vi "BMU参数读取-Auto.vi"(7 "Socket":dbl, 8 "CAN端口":u16(ring), 9 "设备索引号":u16(ring), 10 "CAN卡类型":u32(ring)=21, 11 "从板号":u8=1) -> (3 "成功?":bool)   [LabVIEW 2013] (continued)
            }
          }
          event "DO1": Value Change {
            n4242 = event-data() -> ("NewVal"=w6074:bool)  [unwired: 6 out]
            n4243 = stacked-sequence {
              tunnel: w6074 -> [_ w6087 _]
              frame #0 {
                w6077 = FALSE ("清BUFF")
                n4244 = local write "继电器超时处理"(FALSE ("继电器超时处理")) -> ()
                n4245 = local write "清BUFF"(w6077) -> ()
                n4246 = local write "正级继电器 9"(w6077) -> ()
                n4247 = local write "主从选择"(enum32{"主板", "从板"}."主板" ("主从选择")) -> ()
              }
              frame #1 {
                n4248 = case shown="真" w6087 {
                  selector: w6087 -> [w6102 w6122]
                  tunnel: [w6101 w6121] -> w6086
                  tunnel: [w6089 w6109] -> w6081
                  frame False {
                    w6097 = 256.0 ("y")
                    w6089 = u32 2 ("命令序号")
                    w6101 = u8 192 ("命令")
                    n4249 = local read "动作保持时间"() -> (w6098:dbl)
                    n4250 = Quotient & Remainder(x=w6098, y=w6097) -> (x-y*floor(x/y)=w6090:dbl, floor(x/y)=w6094:dbl)
                    n4251 = Quotient & Remainder(x=w6094, y=w6097) -> (x-y*floor(x/y)=w6091:dbl, floor(x/y)=w6095:dbl)
                    n4252 = Quotient & Remainder(x=w6095, y=w6097) -> (x-y*floor(x/y)=w6092:dbl, floor(x/y)=w6096:dbl)
                    n4253 = local read "设备索引号"() -> (w6106:u16)
                    n4254 = local read "CAN卡类型"() -> (w6107:u32)
                    n4255 = local read "CAN端口"() -> (w6105:u16)
                    n4256 = Boolean To (0,1)(Boolean=w6102) -> (0, 1=w6099:i16)
                    n4257 = Quotient & Remainder(x=w6096, y=w6097) -> (x-y*floor(x/y)=w6093:dbl)  [unwired: 1 out]
                    n4258 = Build Array(i16 1 ("元素"), w6099, w6093, w6092, w6091, w6090, 0.0 ("元素")) -> (w6103:dbl[])
                    n4259 = call "多帧发送机制(EV05).vi"("can卡类型"=w6107, "设备索引号"=w6106, "CAN端口"=w6105, "命令"=w6101, "板号"=u8 0, "命令序号"=w6089, "输入数据"=w6103) -> ()  [unwired: 2 in, 11 out]
                  }
                  frame True {
                    w6117 = 256.0 ("y")
                    w6109 = u32 2 ("命令序号")
                    w6121 = u8 192 ("命令")
                    n4260 = local read "动作保持时间"() -> (w6118:dbl)
                    n4261 = Quotient & Remainder(x=w6118, y=w6117) -> (x-y*floor(x/y)=w6110:dbl, floor(x/y)=w6114:dbl)
                    n4262 = Quotient & Remainder(x=w6114, y=w6117) -> (x-y*floor(x/y)=w6111:dbl, floor(x/y)=w6115:dbl)
                    n4263 = Quotient & Remainder(x=w6115, y=w6117) -> (x-y*floor(x/y)=w6112:dbl, floor(x/y)=w6116:dbl)
                    n4264 = local read "设备索引号"() -> (w6126:u16)
                    n4265 = local read "CAN卡类型"() -> (w6127:u32)
                    n4266 = local read "CAN端口"() -> (w6125:u16)
                    n4267 = Boolean To (0,1)(Boolean=w6122) -> (0, 1=w6119:i16)
                    n4268 = Quotient & Remainder(x=w6116, y=w6117) -> (x-y*floor(x/y)=w6113:dbl)  [unwired: 1 out]
                    n4269 = Build Array(i16 1 ("元素"), w6119, w6113, w6112, w6111, w6110, 0.0 ("元素")) -> (w6123:dbl[])
                    n4270 = call "多帧发送机制(EV05).vi"("can卡类型"=w6127, "设备索引号"=w6126, "CAN端口"=w6125, "命令"=w6121, "板号"=u8 0, "命令序号"=w6109, "输入数据"=w6123) -> ()  [unwired: 2 in, 11 out]
                  }
                }
                n4271 = local write "命令序号"(w6081) -> ()
                n4272 = local write "命令"(w6086) -> ()
                n4273 = local write "控制1"(TRUE ("控制1")) -> ()
                n4274 = local write "写?"(FALSE ("写?")) -> ()
                n4275 = local write "消除"(TRUE ("消除")) -> ()
                n4276 = global write "EV05全局变量1.vi" "流控帧 2"(TRUE ("流控帧 2")) -> ()
                n4277 = global write "EV05全局变量1.vi" "流控帧"(FALSE ("流控帧")) -> ()
              }
              frame #2 {
                n4278 = flat-sequence {
                  tunnel: [w6129] -> w6128
                  tunnel: w6128 -> [w6136]
                  frame #0 {
                    n4279 = while {
                      tunnel: [w6130] -> w6129
                      i -> [w6134]
                      stop <- w6131 stop-if-true
                      n4280 = local read "继电器超时处理"() -> (w6130:bool)
                      n4281 = Greater Or Equal?(x=w6134, y=20) -> (x >= y?=w6132:bool)
                      n4282 = Wait Until Next ms Multiple(millisecond multiple=u32 100 ("毫秒倍数")) -> ()  [unwired: 1 out]
                      n4283 = Or(x=w6130, y=w6132) -> (x .or. y?=w6131:bool)
                    }
                  }
                  frame #1 {
                    n4284 = case shown="假" w6136 {
                      frame False {
                        n4285 = local read "DO1"() -> (w6138:bool)
                        n4286 = Not(x=w6138) -> (.not. x?=w6137:bool)
                        n4287 = local write "DO1"(w6137) -> ()
                        n4288 = One Button Dialog(message="DO控制处理超时" ("消息"), button name ("OK")="是" ("按钮名称（“确定”）")) -> ()  [unwired: 1 out]
                      }
                      frame True {
                      }
                    }
                  }
                }
              }
            }
          }
          event "DO2": Value Change {
            n4289 = event-data() -> ("NewVal"=w6141:bool)  [unwired: 6 out]
            n4290 = stacked-sequence {
              tunnel: w6141 -> [_ w6154 _]
              frame #0 {
                w6144 = FALSE ("清BUFF")
                n4291 = local write "继电器超时处理"(FALSE ("继电器超时处理")) -> ()
                n4292 = local write "主从选择"(enum32{"主板", "从板"}."主板" ("主从选择")) -> ()
                n4293 = local write "清BUFF"(w6144) -> ()
                n4294 = local write "正级继电器 10"(w6144) -> ()
              }
              frame #1 {
                n4295 = case shown="真" w6154 {
                  selector: w6154 -> [w6169 w6189]
                  tunnel: [w6168 w6188] -> w6153
                  tunnel: [w6156 w6176] -> w6148
                  frame False {
                    w6164 = 256.0 ("y")
                    w6156 = u32 2 ("命令序号")
                    w6168 = u8 192 ("命令")
                    n4296 = local read "动作保持时间"() -> (w6165:dbl)
                    n4297 = Quotient & Remainder(x=w6165, y=w6164) -> (x-y*floor(x/y)=w6157:dbl, floor(x/y)=w6161:dbl)
                    n4298 = Quotient & Remainder(x=w6161, y=w6164) -> (x-y*floor(x/y)=w6158:dbl, floor(x/y)=w6162:dbl)
                    n4299 = Quotient & Remainder(x=w6162, y=w6164) -> (x-y*floor(x/y)=w6159:dbl, floor(x/y)=w6163:dbl)
                    n4300 = local read "设备索引号"() -> (w6173:u16)
                    n4301 = local read "CAN卡类型"() -> (w6174:u32)
                    n4302 = local read "CAN端口"() -> (w6172:u16)
                    n4303 = Boolean To (0,1)(Boolean=w6169) -> (0, 1=w6166:i16)
                    n4304 = Quotient & Remainder(x=w6163, y=w6164) -> (x-y*floor(x/y)=w6160:dbl)  [unwired: 1 out]
                    n4305 = Build Array(i16 2 ("元素"), w6166, w6160, w6159, w6158, w6157, 0.0 ("元素")) -> (w6170:dbl[])
                    n4306 = call "多帧发送机制(EV05).vi"("can卡类型"=w6174, "设备索引号"=w6173, "CAN端口"=w6172, "命令"=w6168, "板号"=u8 0, "命令序号"=w6156, "输入数据"=w6170) -> ()  [unwired: 2 in, 11 out]
                  }
                  frame True {
                    w6184 = 256.0 ("y")
                    w6176 = u32 2 ("命令序号")
                    w6188 = u8 192 ("命令")
                    n4307 = local read "动作保持时间"() -> (w6185:dbl)
                    n4308 = Quotient & Remainder(x=w6185, y=w6184) -> (x-y*floor(x/y)=w6177:dbl, floor(x/y)=w6181:dbl)
                    n4309 = Quotient & Remainder(x=w6181, y=w6184) -> (x-y*floor(x/y)=w6178:dbl, floor(x/y)=w6182:dbl)
                    n4310 = Quotient & Remainder(x=w6182, y=w6184) -> (x-y*floor(x/y)=w6179:dbl, floor(x/y)=w6183:dbl)
                    n4311 = local read "设备索引号"() -> (w6193:u16)
                    n4312 = local read "CAN卡类型"() -> (w6194:u32)
                    n4313 = local read "CAN端口"() -> (w6192:u16)
                    n4314 = Boolean To (0,1)(Boolean=w6189) -> (0, 1=w6186:i16)
                    n4315 = Quotient & Remainder(x=w6183, y=w6184) -> (x-y*floor(x/y)=w6180:dbl)  [unwired: 1 out]
                    n4316 = Build Array(i16 2 ("元素"), w6186, w6180, w6179, w6178, w6177, 0.0 ("元素")) -> (w6190:dbl[])
                    n4317 = call "多帧发送机制(EV05).vi"("can卡类型"=w6194, "设备索引号"=w6193, "CAN端口"=w6192, "命令"=w6188, "板号"=u8 0, "命令序号"=w6176, "输入数据"=w6190) -> ()  [unwired: 2 in, 11 out]
                  }
                }
                n4318 = local write "命令序号"(w6148) -> ()
                n4319 = local write "命令"(w6153) -> ()
                n4320 = local write "控制1"(TRUE ("控制1")) -> ()
                n4321 = local write "写?"(FALSE ("写?")) -> ()
                n4322 = local write "消除"(TRUE ("消除")) -> ()
                n4323 = global write "EV05全局变量1.vi" "流控帧 2"(TRUE ("流控帧 2")) -> ()
                n4324 = global write "EV05全局变量1.vi" "流控帧"(FALSE ("流控帧")) -> ()
              }
              frame #2 {
                n4325 = flat-sequence {
                  tunnel: [w6196] -> w6195
                  tunnel: w6195 -> [w6203]
                  frame #0 {
                    n4326 = while {
                      tunnel: [w6197] -> w6196
                      i -> [w6201]
                      stop <- w6198 stop-if-true
                      n4327 = local read "继电器超时处理"() -> (w6197:bool)
                      n4328 = Greater Or Equal?(x=w6201, y=20) -> (x >= y?=w6199:bool)
                      n4329 = Wait Until Next ms Multiple(millisecond multiple=u32 100 ("毫秒倍数")) -> ()  [unwired: 1 out]
                      n4330 = Or(x=w6197, y=w6199) -> (x .or. y?=w6198:bool)
                    }
                  }
                  frame #1 {
                    n4331 = case shown="假" w6203 {
                      frame False {
                        n4332 = local read "DO2"() -> (w6205:bool)
                        n4333 = Not(x=w6205) -> (.not. x?=w6204:bool)
                        n4334 = local write "DO2"(w6204) -> ()
                        n4335 = One Button Dialog(message="DO控制处理超时" ("消息"), button name ("OK")="是" ("按钮名称（“确定”）")) -> ()  [unwired: 1 out]
                      }
                      frame True {
                      }
                    }
                  }
                }
              }
            }
          }
          event "DO1 2": Value Change {
            n4336 = event-data() -> ("NewVal"=w6208:bool)  [unwired: 6 out]
            n4337 = stacked-sequence {
              tunnel: w6208 -> [_ w6222 _]
              frame #0 {
                w6211 = FALSE ("继电器超时处理")
                n4338 = local write "继电器超时处理"(w6211) -> ()
                n4339 = local write "正级继电器 11"(w6211) -> ()
                n4340 = local write "主从选择"(enum32{"主板", "从板"}."从板" ("主从选择")) -> ()
              }
              frame #1 {
                n4341 = case shown="假" w6222 {
                  selector: w6222 -> [w6237 w6257]
                  tunnel: [w6236 w6256] -> w6221
                  tunnel: [w6235 w6255] -> w6215
                  tunnel: [w6224 w6244] -> w6216
                  frame True {
                    w6232 = 256.0 ("y")
                    w6224 = u32 2 ("命令序号")
                    w6236 = u8 192 ("命令")
                    n4342 = local read "动作保持时间"() -> (w6233:dbl)
                    n4343 = Quotient & Remainder(x=w6233, y=w6232) -> (x-y*floor(x/y)=w6225:dbl, floor(x/y)=w6229:dbl)
                    n4344 = Quotient & Remainder(x=w6229, y=w6232) -> (x-y*floor(x/y)=w6226:dbl, floor(x/y)=w6230:dbl)
                    n4345 = Quotient & Remainder(x=w6230, y=w6232) -> (x-y*floor(x/y)=w6227:dbl, floor(x/y)=w6231:dbl)
                    n4346 = Quotient & Remainder(x=w6231, y=w6232) -> (x-y*floor(x/y)=w6228:dbl)  [unwired: 1 out]
                    n4347 = Boolean To (0,1)(Boolean=w6237) -> (0, 1=w6234:i16)
                    n4348 = local read "设备索引号"() -> (w6241:u16)
                    n4349 = local read "CAN卡类型"() -> (w6242:u32)
                    n4350 = local read "从板板号"() -> (w6235:u8)
                    n4351 = local read "CAN端口"() -> (w6240:u16)
                    n4352 = Build Array(i16 3 ("元素"), w6234, w6228, w6227, w6226, w6225, 0.0 ("元素")) -> (w6239:dbl[])
                    n4353 = call "多帧发送机制(EV05).vi"("can卡类型"=w6242, "设备索引号"=w6241, "CAN端口"=w6240, "命令"=w6236, "板号"=w6235, "命令序号"=w6224, "输入数据"=w6239) -> ()  [unwired: 2 in, 11 out]
                  }
                  frame False {
                    w6252 = 256.0 ("y")
                    w6244 = u32 2 ("命令序号")
                    w6256 = u8 192 ("命令")
                    n4354 = local read "动作保持时间"() -> (w6253:dbl)
                    n4355 = Quotient & Remainder(x=w6253, y=w6252) -> (x-y*floor(x/y)=w6245:dbl, floor(x/y)=w6249:dbl)
                    n4356 = Quotient & Remainder(x=w6249, y=w6252) -> (x-y*floor(x/y)=w6246:dbl, floor(x/y)=w6250:dbl)
                    n4357 = Quotient & Remainder(x=w6250, y=w6252) -> (x-y*floor(x/y)=w6247:dbl, floor(x/y)=w6251:dbl)
                    n4358 = Quotient & Remainder(x=w6251, y=w6252) -> (x-y*floor(x/y)=w6248:dbl)  [unwired: 1 out]
                    n4359 = Boolean To (0,1)(Boolean=w6257) -> (0, 1=w6254:i16)
                    n4360 = local read "设备索引号"() -> (w6261:u16)
                    n4361 = local read "CAN卡类型"() -> (w6262:u32)
                    n4362 = local read "从板板号"() -> (w6255:u8)
                    n4363 = local read "CAN端口"() -> (w6260:u16)
                    n4364 = Build Array(i16 1 ("元素"), w6254, w6248, w6247, w6246, w6245, 0.0 ("元素")) -> (w6259:dbl[])
                    n4365 = call "多帧发送机制(EV05).vi"("can卡类型"=w6262, "设备索引号"=w6261, "CAN端口"=w6260, "命令"=w6256, "板号"=w6255, "命令序号"=w6244, "输入数据"=w6259) -> ()  [unwired: 2 in, 11 out]
                  }
                }
                n4366 = local write "从板板号"(w6215) -> ()
                n4367 = local write "命令序号"(w6216) -> ()
                n4368 = local write "命令"(w6221) -> ()
                n4369 = local write "清BUFF"(FALSE ("清BUFF")) -> ()
                n4370 = local write "写?"(FALSE ("写?")) -> ()
                n4371 = local write "控制1"(TRUE ("控制1")) -> ()
                n4372 = global write "EV05全局变量1.vi" "流控帧"(FALSE ("流控帧")) -> ()
                n4373 = global write "EV05全局变量1.vi" "流控帧 2"(TRUE ("流控帧 2")) -> ()
                n4374 = local write "消除"(TRUE ("消除")) -> ()
              }
              frame #2 {
                n4375 = flat-sequence {
                  tunnel: [w6264] -> w6263
                  tunnel: w6263 -> [w6271]
                  frame #0 {
                    n4376 = while {
                      tunnel: [w6265] -> w6264
                      i -> [w6269]
                      stop <- w6266 stop-if-true
                      n4377 = local read "继电器超时处理"() -> (w6265:bool)
                      n4378 = Greater Or Equal?(x=w6269, y=20) -> (x >= y?=w6267:bool)
                      n4379 = Wait Until Next ms Multiple(millisecond multiple=u32 100 ("毫秒倍数")) -> ()  [unwired: 1 out]
                      n4380 = Or(x=w6265, y=w6267) -> (x .or. y?=w6266:bool)
                    }
                  }
                  frame #1 {
                    n4381 = case shown="假" w6271 {
                      frame False {
                        n4382 = local read "DO1 2"() -> (w6273:bool)
                        n4383 = Not(x=w6273) -> (.not. x?=w6272:bool)
                        n4384 = local write "DO1 2"(w6272) -> ()
                        n4385 = One Button Dialog(message="DO控制处理超时" ("消息"), button name ("OK")="是" ("按钮名称（“确定”）")) -> ()  [unwired: 1 out]
                      }
                      frame True {
                      }
                    }
                  }
                }
              }
            }
          }
          event "读取转换为写入": Value Change {
            n4386 = event-data() -> ("NewVal"=w6276:bool)  [unwired: 6 out]
            n4387 = case shown="真" w6276 {
              tunnel: w6280 -> [w6282 w6287]
              tunnel: [w6282 w6286] -> w6279
              tunnel: w6278 -> [w6281 w6285]
              tunnel: [w6281 w6284] -> w6277
              frame False {
              }
              frame True {
                n4388 = Enqueue Element(queue=w6287, element="读取转换为写入", error in (no error)=w6285) -> (queue out=w6286:refnum<queue>, error out=w6284:errorcluster)  [unwired: 2 out]
              }
            }
          }
          event "读取故障详细状态": Value Change {
            n4389 = event-data() -> ("NewVal"=w6292:bool)  [unwired: 5 out]
            n4390 = case shown="真" w6292 {
              tunnel: w6291 -> [w6294 w6307]
              tunnel: w6290 -> [w6293 w6306]
              tunnel: [w6294 w6305] -> w6289
              tunnel: [w6293 w6304] -> w6288
              frame False {
              }
              frame True {
                n4391 = disable-structure shown="启用" {
                  disable-tunnel: [w6316 TRUE ("发送成功")] -> w6303
                  frame Disabled {
                    n4392 = local read "主从选择"() -> (w6308:enum32{"主板", "从板"})
                    n4393 = case shown="\"主板\", 默认" w6308 {
                      tunnel: [0.0 ("FUNC") w6318] -> w6313
                      frame "主板", Default {
                      }
                      frame "从板" {
                        n4394 = local read "从板号"() -> (w6318:u8)
                      }
                    }
                    n4395 = local read "设备索引号"() -> (w6310:u16)
                    n4396 = local read "CAN卡类型"() -> (w6311:u32)
                    n4397 = local read "CAN端口"() -> (w6309:u16)
                    n4398 = call "标定授权发送.vi"("CAN卡类型"=w6311, "解锁类型"=enum16{"读取", "写", "下载"}."写", "设备索引号"=w6310, "CAN端口"=w6309, "是否连接"=TRUE, "板选择"=0, "FUNC"=w6313) -> ("发送成功"=w6316:bool)  [unwired: 8 out]
                  }
                  frame Enabled {
                  }
                }
                n4399 = case shown="真" w6303 {
                  tunnel: w6307 -> [w6321 w6326]
                  tunnel: w6306 -> [w6320 w6325]
                  tunnel: [w6321 w6323] -> w6305
                  tunnel: [w6320 w6322] -> w6304
                  frame False {
                  }
                  frame True {
                    n4400 = Enqueue Element(queue=w6326, element="读取故障状态" ("元素"), error in (no error)=w6325) -> (queue out=w6323:refnum<queue>, error out=w6322:errorcluster)  [unwired: 2 out]
                  }
                }
                n4401 = local write "电池故障"(string[][] []) -> ()
                n4402 = global write "EV05全局变量1.vi" "流控帧 2"(TRUE ("流控帧")) -> ()
                n4403 = local write "写?"(FALSE ("写?")) -> ()
                n4404 = local write "控制1"(TRUE ("控制1")) -> ()
                n4405 = local write "消除"(TRUE ("消除")) -> ()
                n4406 = local write "清BUFF"(FALSE ("清BUFF")) -> ()
                n4407 = global write "EV05全局变量1.vi" "流控帧"(FALSE ("流控帧")) -> ()
                n4408 = call <vilib>:"Set Busy.vi"("disable click? (T)"=FALSE) -> ()  [unwired: 3 in, 8 out]
              }
            }
          }
          event "项目软本读取": Value Change {
            n4409 = event-data() -> ("NewVal"=w6331:bool)  [unwired: 5 out]
            n4410 = case shown="真" w6331 {
              tunnel: w6330 -> [w6333 w6338]
              tunnel: w6329 -> [w6332 w6337]
              tunnel: [w6333 w6336] -> w6328
              tunnel: [w6332 w6335] -> w6327
              frame False {
              }
              frame True {
                n4411 = stacked-sequence {
                  tunnel: [w6341] -> _
                  frame #0 {
                    w6341 = FALSE ("disable click? (T)")
                    w6344 = FALSE ("写?")
                    n4412 = local write "写?"(w6344) -> ()
                    n4413 = global write "EV05全局变量1.vi" "写入超时"(w6344) -> ()
                    n4414 = local write "项目软件版本号"(" " ("项目软件版本号")) -> ()
                    n4415 = global write "EV05全局变量1.vi" "流控帧"(FALSE ("流控帧")) -> ()
                    n4416 = local write "主从选择"(enum32{"主板", "从板"}."主板" ("主从选择")) -> ()
                    n4417 = call <vilib>:"Set Busy.vi"("disable click? (T)"=w6341) -> ()  [unwired: 3 in, 8 out]
                    n4418 = local write "清BUFF"(FALSE ("清BUFF")) -> ()
                    n4419 = property on="保存版本信息" class="Bool (严格)"("Visible"=TRUE ("可见")) -> ()  [unwired: 2 in, 2 out]
                    n4420 = global write "EV05全局变量1.vi" "流控帧 2"(TRUE ("流控帧 2")) -> ()
                    n4421 = local write "控制1"(TRUE ("控制1")) -> ()
                    n4422 = local write "消除"(TRUE ("消除")) -> ()
                  }
                }
                n4423 = Enqueue Element(queue=w6338, element="项目软件版本读取" ("元素"), error in (no error)=w6337) -> (queue out=w6336:refnum<queue>, error out=w6335:errorcluster)  [unwired: 2 out]
              }
            }
          }
          event "读硬件版本号": Value Change {
            n4424 = event-data() -> ("NewVal"=w6353:bool)  [unwired: 5 out]
            n4425 = case shown="真" w6353 {
              tunnel: w6352 -> [w6355 w6362]
              tunnel: w6351 -> [w6354 w6361]
              tunnel: [w6355 w6360] -> w6350
              tunnel: [w6354 w6359] -> w6349
              frame False {
              }
              frame True {
                n4426 = global read "EV05全局变量1.vi" "授权功能"() -> (w6357:bool)
                n4427 = case shown="真" w6357 {
                  tunnel: [TRUE ("发送成功") w6381] -> w6358
                  frame False {
                  }
                  frame True {
                    n4428 = local read "设备索引号"() -> (w6376:u16)
                    n4429 = local read "CAN卡类型"() -> (w6377:u32)
                    n4430 = local read "CAN端口"() -> (w6375:u16)
                    n4431 = call "标定授权发送.vi"("CAN卡类型"=w6377, "解锁类型"=enum16{"读取", "写", "下载"}."读取", "设备索引号"=w6376, "CAN端口"=w6375, "是否连接"=TRUE, "板选择"=0, "FUNC"=u32 0) -> ("发送成功"=w6381:bool)  [unwired: 8 in]
                  }
                }
                n4432 = stacked-sequence {
                  tunnel: [w6365] -> w6356
                  frame #0 {
                    w6365 = TRUE ("控制1")
                    w6369 = FALSE ("写?")
                    n4433 = local write "写?"(w6369) -> ()
                    n4434 = global write "EV05全局变量1.vi" "写入超时"(w6369) -> ()
                    n4435 = call <vilib>:"Set Busy.vi"("disable click? (T)"=FALSE) -> ()  [unwired: 3 in, 8 out]
                    n4436 = local write "硬件版本号"("" ("硬件版本号")) -> ()
                    n4437 = property on="保存版本信息" class="Bool (严格)"("Visible"=TRUE ("可见")) -> ()  [unwired: 2 in, 2 out]
                    n4438 = local write "主从选择"(enum32{"主板", "从板"}."主板" ("主从选择")) -> ()
                    n4439 = local write "控制1"(w6365) -> ()
                    n4440 = local write "清BUFF"(FALSE ("清BUFF")) -> ()
                    n4441 = global write "EV05全局变量1.vi" "流控帧 2"(TRUE ("流控帧 2")) -> ()
                    n4442 = local write "消除"(TRUE ("消除")) -> ()
                    n4443 = global write "EV05全局变量1.vi" "流控帧"(FALSE ("流控帧")) -> ()
                  }
                }
                n4444 = case shown="真" w6358 {
                  tunnel: w6362 -> [w6383 w6388]
                  tunnel: w6361 -> [w6382 w6387]
                  tunnel: [w6383 w6385] -> w6360
                  tunnel: [w6382 w6384] -> w6359
                  tunnel: w6356 -> [_ _]
                  frame False {
                  }
                  frame True {
                    n4445 = Enqueue Element(queue=w6388, element="硬件版本读取" ("元素"), error in (no error)=w6387) -> (queue out=w6385:refnum<queue>, error out=w6384:errorcluster)  [unwired: 2 out]
                  }
                }
              }
            }
          }
          event "平台软件版本读取": Value Change {
            n4446 = event-data() -> ("NewVal"=w6393:bool)  [unwired: 5 out]
            n4447 = case shown="真" w6393 {
              tunnel: w6392 -> [w6395 w6400]
              tunnel: w6391 -> [w6394 w6399]
              tunnel: [w6395 w6398] -> w6390
              tunnel: [w6394 w6397] -> w6389
              frame False {
              }
              frame True {
                n4448 = stacked-sequence {
                  tunnel: [w6403] -> _
                  frame #0 {
                    w6403 = TRUE ("控制1")
                    w6407 = FALSE ("写?")
                    n4449 = call <vilib>:"Set Busy.vi"("disable click? (T)"=FALSE) -> ()  [unwired: 3 in, 8 out]
                    n4450 = local write "写?"(w6407) -> ()
                    n4451 = global write "EV05全局变量1.vi" "写入超时"(w6407) -> ()
                    n4452 = local write "平台软件版本号"(" " ("平台软件版本号")) -> ()
                    n4453 = local write "控制1"(w6403) -> ()
                    n4454 = local write "消除"(TRUE ("消除")) -> ()
                    n4455 = property on="保存版本信息" class="Bool (严格)"("Visible"=TRUE ("可见")) -> ()  [unwired: 2 in, 2 out]
                    n4456 = global write "EV05全局变量1.vi" "流控帧 2"(TRUE ("流控帧 2")) -> ()
                    n4457 = local write "主从选择"(enum32{"主板", "从板"}."主板" ("主从选择")) -> ()
                    n4458 = local write "清BUFF"(FALSE ("清BUFF")) -> ()
                    n4459 = global write "EV05全局变量1.vi" "流控帧"(FALSE ("流控帧")) -> ()
                  }
                }
                n4460 = Enqueue Element(queue=w6400, element="平台软件版本读取" ("元素"), error in (no error)=w6399) -> (queue out=w6398:refnum<queue>, error out=w6397:errorcluster)  [unwired: 2 out]
              }
            }
          }
          event "模块版本读取": Value Change {
            n4461 = event-data() -> ("NewVal"=w6415:bool)  [unwired: 5 out]
            n4462 = case shown="真" w6415 {
              tunnel: w6414 -> [w6417 w6424]
              tunnel: w6413 -> [w6416 w6423]
              tunnel: [w6417 w6422] -> w6412
              tunnel: [w6416 w6421] -> w6411
              frame False {
              }
              frame True {
                n4463 = global read "EV05全局变量1.vi" "授权功能"() -> (w6419:bool)
                n4464 = case shown="假" w6419 {
                  tunnel: [TRUE ("发送成功") w6442] -> w6420
                  frame False {
                  }
                  frame True {
                    n4465 = local read "设备索引号"() -> (w6437:u16)
                    n4466 = local read "CAN卡类型"() -> (w6438:u32)
                    n4467 = local read "CAN端口"() -> (w6436:u16)
                    n4468 = call "标定授权发送.vi"("CAN卡类型"=w6438, "解锁类型"=enum16{"读取", "写", "下载"}."读取", "设备索引号"=w6437, "CAN端口"=w6436, "是否连接"=TRUE, "板选择"=0, "FUNC"=u32 0) -> ("发送成功"=w6442:bool)  [unwired: 8 out]
                  }
                }
                n4469 = stacked-sequence {
                  tunnel: [w6427] -> w6418
                  frame #0 {
                    w6427 = TRUE ("控制1")
                    w6430 = FALSE ("写?")
                    n4470 = call <vilib>:"Set Busy.vi"("disable click? (T)"=FALSE) -> ()  [unwired: 3 in, 8 out]
                    n4471 = local write "写?"(w6430) -> ()
                    n4472 = global write "EV05全局变量1.vi" "写入超时"(w6430) -> ()
                    n4473 = local write "主从选择"(enum32{"主板", "从板"}."主板" ("主从选择")) -> ()
                    n4474 = local write "清BUFF"(FALSE ("清BUFF")) -> ()
                    n4475 = property on="保存版本信息" class="Bool (严格)"("Visible"=TRUE ("可见")) -> ()  [unwired: 2 in, 2 out]
                    n4476 = global write "EV05全局变量1.vi" "流控帧 2"(TRUE ("流控帧 2")) -> ()
                    n4477 = local write "控制1"(w6427) -> ()
                    n4478 = local write "消除"(TRUE ("消除")) -> ()
                    n4479 = global write "EV05全局变量1.vi" "流控帧"(FALSE ("流控帧")) -> ()
                  }
                }
                n4480 = case shown="真" w6420 {
                  tunnel: w6424 -> [w6444 w6449]
                  tunnel: w6423 -> [w6443 w6448]
                  tunnel: [w6444 w6446] -> w6422
                  tunnel: [w6443 w6445] -> w6421
                  tunnel: w6418 -> [_ _]
                  frame False {
                  }
                  frame True {
                    n4481 = Enqueue Element(queue=w6449, element="模块软件版本读取" ("元素"), error in (no error)=w6448) -> (queue out=w6446:refnum<queue>, error out=w6445:errorcluster)  [unwired: 2 out]
                  }
                }
              }
            }
          }
          event "保存版本信息": Value Change {
            n4482 = event-data() -> ("NewVal"=w6450:bool)  [unwired: 6 out]
            n4483 = case shown="真" w6450 {
              frame False {
              }
              frame True {
                n4484 = stacked-sequence {
                  seq-local: [w6454 _] -> [_ w6456]
                  seq-local: [w6453 _] -> [_ w6455]
                  frame #0 {
                    n4485 = call "请输入从板个数"() -> ("从板个数"=w6454:dbl, "确定"=w6453:bool)  [unwired: 17 in, 1 out]
                  }
                  frame #1 {
                    n4486 = case shown="真" w6455 {
                      tunnel: w6456 -> [_ w6459]
                      frame False {
                      }
                      frame True {
                        n4487 = call <vilib>:"Application Directory.vi"() -> ("Application Directory"=w6471:path)
                        n4488 = Build Path(base path=w6471, name or relative path="SaveData" ("名称或相对路径")) -> (appended path=w6469:path)
                        n4489 = local read "模块版本名称"() -> (w6464:string[][])
                        n4490 = local read "项目软件版本"() -> (w6461:string[])
                        n4491 = local read "模块版本值"() -> (w6463:string[][])
                        n4492 = local read "平台软件版本"() -> (w6460:string[])
                        n4493 = local read "模块个数"() -> (w6457:u8[])
                        n4494 = local read "硬件版本"() -> (w6462:string[])
                        n4495 = call "文件对话框3"("start path"=w6469, "prompt"="选择要保存数据的位置", "default name"="BMS版本信息.txt") -> ("selected path"=w6465:path, "cancelled"=w6466:bool)  [unwired: 9 in, 2 out]
                        n4496 = Increment(x=w6459) -> (x+1=w6458:dbl)
                        n4497 = for {
                          N: w6458 -> [_]
                          tunnel: w6466 -> [w6487]
                          tunnel: w6465 -> [w6486]
                          tunnel: w6464 -> [w6476] mode=indexing
                          tunnel: w6463 -> [w6474] mode=indexing
                          tunnel: w6462 -> [w6481] mode=indexing
                          tunnel: w6461 -> [w6480] mode=indexing
                          tunnel: w6460 -> [w6479] mode=indexing
                          tunnel: w6457 -> [w6472] mode=indexing
                          i -> [w6478]
                          w6484 = ""
                          w6491 = 0 ("索引")
                          n4498 = case shown="0, 默认" w6478 {
                            selector: w6478 -> [_ w6505]
                            tunnel: ["主板版本信息" w6506] -> w6496
                            tunnel: [FALSE TRUE] -> w6482
                            frame 0, Default {
                            }
                            frame 1.. {
                              n4499 = Number To Decimal String(number=w6505) -> (decimal integer string=w6504:string)  [unwired: 1 in]
                              n4500 = Concatenate Strings("从板", w6504, "版本信息") -> (w6506:string)
                            }
                          }
                          n4501 = Increment(x=w6472) -> (x+1=w6473:u8)
                          n4502 = Array Subset(array=w6476, length=w6473) -> (w6477:string[])  [unwired: 1 in]
                          n4503 = Array Subset(array=w6474, length=w6473) -> (w6475:string[])  [unwired: 1 in]
                          n4504 = Build Array(w6484, w6479, w6480, w6481, w6484) -> (w6490:string[])
                          n4505 = Build Array(w6496, "平台软件版本号", "项目软件版本号", "硬件版本号", "模块版本号") -> (w6492:string[])
                          n4506 = Insert Into Array(array=w6477, index=w6491, new element=w6492) -> (w6489:string[])
                          n4507 = Insert Into Array(array=w6475, index=w6491, new element=w6490) -> (w6488:string[])
                          n4508 = Build Array(w6489, w6488) -> (w6485:string[][])
                          n4509 = case shown="假" w6487 {
                            tunnel: w6486 -> [w6500 _]
                            tunnel: w6485 -> [w6499 _]
                            tunnel: w6482 -> [w6497 _]
                            frame False {
                              n4510 = call-poly <vilib>:"Write To Spreadsheet File.vi"("transpose? (no:F)"=TRUE, "append to file? (new file:F)"=w6497, "2D data"=w6499, "file path (dialog if empty)"=w6500) -> ()  [unwired: 4 in, 1 out]
                            }
                            frame True {
                            }
                          }
                        }
                      }
                    }
                  }
                }
              }
            }
          }
          event "单个写入": Value Change {
            n4511 = event-data() -> ("NewVal"=w6513:bool)  [unwired: 5 out]
            n4512 = case shown="真" w6513 {
              tunnel: w6512 -> [w6515 w6522]
              tunnel: w6511 -> [w6514 w6521]
              tunnel: [w6515 w6520] -> w6510
              tunnel: [w6514 w6519] -> w6509
              frame False {
              }
              frame True {
                w6517 = FALSE ("流控帧")
                w6516 = TRUE ("流控帧 2")
                n4513 = disable-structure shown="禁用" {
                  disable-tunnel: [w6531 TRUE ("发送成功")] -> w6518
                  frame Disabled {
                    n4514 = local read "主从选择"() -> (w6523:enum32{"主板", "从板"})
                    n4515 = case shown="\"主板\", 默认" w6523 {
                      tunnel: [0.0 ("FUNC") w6533] -> w6528
                      frame "主板", Default {
                      }
                      frame "从板" {
                        n4516 = local read "从板号"() -> (w6533:u8)
                      }
                    }
                    n4517 = local read "设备索引号"() -> (w6525:u16)
                    n4518 = local read "CAN卡类型"() -> (w6526:u32)
                    n4519 = local read "CAN端口"() -> (w6524:u16)
                    n4520 = call "标定授权发送.vi"("CAN卡类型"=w6526, "解锁类型"=enum16{"读取", "写", "下载"}."写", "设备索引号"=w6525, "CAN端口"=w6524, "是否连接"=TRUE, "板选择"=0, "FUNC"=w6528) -> ("发送成功"=w6531:bool)  [unwired: 8 out]
                  }
                  frame Enabled {
                  }
                }
                n4521 = case shown="真" w6518 {
                  tunnel: w6522 -> [w6536 w6540]
                  tunnel: w6521 -> [w6535 w6539]
                  tunnel: [w6536 w6542] -> w6520
                  tunnel: [w6535 w6541] -> w6519
                  frame False {
                  }
                  frame True {
                    n4522 = Flush Queue(queue=w6540, error in (no error)=w6539) -> (queue out=w6538:refnum<queue>, error out=w6537:errorcluster)  [unwired: 1 out]
                    n4523 = Enqueue Element(queue=w6538, element="单个写入" ("元素"), error in (no error)=w6537) -> (queue out=w6542:refnum<queue>, error out=w6541:errorcluster)  [unwired: 2 out]
                  }
                }
                n4524 = global write "EV05全局变量1.vi" "读取超时"(w6517) -> ()
                n4525 = global write "EV05全局变量1.vi" "流控帧"(w6517) -> ()
                n4526 = local write "消除"(w6516) -> ()
                n4527 = local write "控制1"(w6516) -> ()
                n4528 = global write "EV05全局变量1.vi" "流控帧 2"(w6516) -> ()
                n4529 = local write "写?"(w6516) -> ()
              }
            }
          }
          event "全部写入": Value Change {
            n4530 = event-data() -> ("NewVal"=w6548:bool)  [unwired: 5 out]
            n4531 = case shown="真" w6548 {
              tunnel: w6547 -> [w6550 w6558]
              tunnel: w6546 -> [w6549 w6557]
              tunnel: [w6550 w6556] -> w6545
              tunnel: [w6549 w6555] -> w6544
              frame False {
              }
              frame True {
                w6552 = FALSE ("流控帧")
                w6551 = TRUE ("流控帧 2")
                n4532 = global read "EV05全局变量1.vi" "授权功能"() -> (w6553:bool)
                n4533 = case shown="真" w6553 {
                  tunnel: [TRUE ("发送成功") w6568] -> w6554
                  frame False {
                  }
                  frame True {
                    n4534 = local read "主从选择"() -> (w6560:enum32{"主板", "从板"})
                    n4535 = case shown="\"从板\"" w6560 {
                      tunnel: [0.0 ("FUNC") w6570] -> w6561
                      frame "主板", Default {
                      }
                      frame "从板" {
                        n4536 = local read "从板号"() -> (w6570:u8)
                      }
                    }
                    n4537 = local read "设备索引号"() -> (w6563:u16)
                    n4538 = local read "CAN卡类型"() -> (w6564:u32)
                    n4539 = local read "CAN端口"() -> (w6562:u16)
                    n4540 = call "标定授权发送.vi"("CAN卡类型"=w6564, "解锁类型"=enum16{"读取", "写", "下载"}."写", "设备索引号"=w6563, "CAN端口"=w6562, "是否连接"=TRUE, "板选择"=0, "FUNC"=w6561) -> ("发送成功"=w6568:bool)  [unwired: 8 out]
                  }
                }
                n4541 = case shown="真" w6554 {
                  tunnel: w6558 -> [w6572 w6576]
                  tunnel: w6557 -> [w6571 w6575]
                  tunnel: [w6572 w6578] -> w6556
                  tunnel: [w6571 w6577] -> w6555
                  frame False {
                  }
                  frame True {
                    n4542 = Flush Queue(queue=w6576, error in (no error)=w6575) -> (queue out=w6574:refnum<queue>, error out=w6573:errorcluster)  [unwired: 1 out]
                    n4543 = Enqueue Element(queue=w6574, element="全部写入" ("元素"), error in (no error)=w6573) -> (queue out=w6578:refnum<queue>, error out=w6577:errorcluster)  [unwired: 1 in, 1 out]
                  }
                }
                n4544 = global write "EV05全局变量1.vi" "读取超时"(w6552) -> ()
                n4545 = global write "EV05全局变量1.vi" "流控帧"(w6552) -> ()
                n4546 = local write "消除"(w6551) -> ()
                n4547 = local write "控制1"(w6551) -> ()
                n4548 = global write "EV05全局变量1.vi" "流控帧 2"(w6551) -> ()
                n4549 = local write "写?"(w6551) -> ()
              }
            }
          }
          event "单个读取": Value Change {
            n4550 = event-data() -> ("NewVal"=w6584:bool)  [unwired: 5 out]
            n4551 = case shown="真" w6584 {
              tunnel: w6583 -> [w6586 w6594]
              tunnel: w6582 -> [w6585 w6593]
              tunnel: [w6586 w6592] -> w6581
              tunnel: [w6585 w6591] -> w6580
              frame False {
              }
              frame True {
                w6587 = FALSE ("流控帧")
                w6588 = TRUE ("流控帧 2")
                n4552 = global read "EV05全局变量1.vi" "授权功能"() -> (w6589:bool)
                n4553 = case shown="假" w6589 {
                  tunnel: [TRUE ("发送成功") w6603] -> w6590
                  frame False {
                  }
                  frame True {
                    n4554 = local read "设备索引号"() -> (w6597:u16)
                    n4555 = local read "CAN卡类型"() -> (w6598:u32)
                    n4556 = local read "CAN端口"() -> (w6596:u16)
                    n4557 = call "标定授权发送.vi"("CAN卡类型"=w6598, "解锁类型"=enum16{"读取", "写", "下载"}."读取", "设备索引号"=w6597, "CAN端口"=w6596, "是否连接"=TRUE, "板选择"=0, "FUNC"=u32 1) -> ("发送成功"=w6603:bool)  [unwired: 8 out]
                  }
                }
                n4558 = case shown="真" w6590 {
                  tunnel: w6594 -> [w6605 w6609]
                  tunnel: w6593 -> [w6604 w6607]
                  tunnel: [w6605 w6611] -> w6592
                  tunnel: [w6604 w6610] -> w6591
                  frame False {
                  }
                  frame True {
                    n4559 = Flush Queue(queue=w6609, error in (no error)=w6607) -> (queue out=w6608:refnum<queue>, error out=w6606:errorcluster)  [unwired: 1 out]
                    n4560 = Enqueue Element(queue=w6608, element="单个读取" ("元素"), error in (no error)=w6606) -> (queue out=w6611:refnum<queue>, error out=w6610:errorcluster)  [unwired: 2 out]
                  }
                }
                n4561 = global write "EV05全局变量1.vi" "写入超时"(w6587) -> ()
                n4562 = global write "EV05全局变量1.vi" "流控帧"(w6587) -> ()
                n4563 = local write "写?"(w6587) -> ()
                n4564 = local write "消除"(w6588) -> ()
                n4565 = local write "控制1"(w6588) -> ()
                n4566 = global write "EV05全局变量1.vi" "流控帧 2"(w6588) -> ()
              }
            }
          }
          event "全部读取": Value Change {
            n4567 = event-data() -> ("NewVal"=w6617:bool)  [unwired: 5 out]
            n4568 = case shown="真" w6617 {
              tunnel: w6616 -> [w6619 w6623]
              tunnel: w6615 -> [w6618 w6622]
              tunnel: [w6619 w6621] -> w6614
              tunnel: [w6618 w6620] -> w6613
              frame False {
              }
              frame True {
                n4569 = stacked-sequence {
                  seq-local: [w6628 _] -> [_ _]
                  seq-local: [w6627 _] -> [_ _]
                  tunnel: w6623 -> [w6630 w6659]
                  tunnel: w6622 -> [w6629 w6658]
                  tunnel: [_ w6663] -> w6621
                  tunnel: [_ w6662] -> w6620
                  frame #0 {
                    w6624 = FALSE ("布尔")
                    n4570 = local read "路径"() -> (w6626:path)
                    n4571 = Empty String/Path?(string/path=w6626) -> (empty?=w6625:bool)
                    n4572 = case shown="假" w6625 {
                      tunnel: w6630 -> [w6637 w6655]
                      tunnel: w6629 -> [w6636 w6654]
                      tunnel: [w6633 w6654] -> w6628
                      tunnel: [w6632 w6655] -> w6627
                      frame False {
                        n4573 = global read "EV05全局变量1.vi" "授权功能"() -> (w6634:bool)
                        n4574 = case shown="真" w6634 {
                          tunnel: [TRUE ("发送成功") w6646] -> w6635
                          frame False {
                          }
                          frame True {
                            n4575 = local read "设备索引号"() -> (w6640:u16)
                            n4576 = local read "CAN卡类型"() -> (w6641:u32)
                            n4577 = local read "CAN端口"() -> (w6639:u16)
                            n4578 = call "标定授权发送.vi"("CAN卡类型"=w6641, "解锁类型"=enum16{"读取", "写", "下载"}."读取", "设备索引号"=w6640, "CAN端口"=w6639, "是否连接"=TRUE, "板选择"=0, "FUNC"=u32 1) -> ("发送成功"=w6646:bool)  [unwired: 8 out]
                          }
                        }
                        n4579 = case shown="真" w6635 {
                          tunnel: w6637 -> [w6648 w6653]
                          tunnel: w6636 -> [w6647 w6652]
                          tunnel: [w6648 w6650] -> w6632
                          tunnel: [w6647 w6649] -> w6633
                          frame False {
                          }
                          frame True {
                            n4580 = Enqueue Element(queue=w6653, element="读配置文件" ("元素"), error in (no error)=w6652) -> (queue out=w6650:refnum<queue>, error out=w6649:errorcluster)  [unwired: 2 out]
                          }
                        }
                        n4581 = Wait Until Next ms Multiple(millisecond multiple=u32 200 ("毫秒倍数")) -> ()  [unwired: 1 out]
                      }
                      frame True {
                      }
                    }
                    n4582 = local write "1 6"(w6624) -> ()
                    n4583 = local write "1 7"(w6624) -> ()
                    n4584 = local write "1 8"(w6624) -> ()
                    n4585 = local write "1 9"(w6624) -> ()
                    n4586 = local write "1 10"(w6624) -> ()
                    n4587 = local write "1 12"(w6624) -> ()
                  }
                  frame #1 {
                    w6656 = FALSE ("流控帧")
                    w6657 = TRUE ("流控帧 2")
                    n4588 = global read "EV05全局变量1.vi" "授权功能"() -> (w6660:bool)
                    n4589 = case shown="假" w6660 {
                      tunnel: [TRUE ("发送成功") w6672] -> w6661
                      frame False {
                      }
                      frame True {
                        n4590 = local read "设备索引号"() -> (w6666:u16)
                        n4591 = local read "CAN卡类型"() -> (w6667:u32)
                        n4592 = local read "CAN端口"() -> (w6665:u16)
                        n4593 = call "标定授权发送.vi"("CAN卡类型"=w6667, "解锁类型"=enum16{"读取", "写", "下载"}."读取", "设备索引号"=w6666, "CAN端口"=w6665, "是否连接"=TRUE, "板选择"=0, "FUNC"=u32 1) -> ("发送成功"=w6672:bool)  [unwired: 8 out]
                      }
                    }
                    n4594 = case shown="真" w6661 {
                      tunnel: w6659 -> [w6674 w6675]
                      tunnel: w6658 -> [w6673 w6678]
                      tunnel: [w6674 w6680] -> w6663
                      tunnel: [w6673 w6679] -> w6662
                      frame False {
                      }
                      frame True {
                        n4595 = Flush Queue(queue=w6675, error in (no error)=w6678) -> (queue out=w6676:refnum<queue>, error out=w6677:errorcluster)  [unwired: 1 out]
                        n4596 = Enqueue Element(queue=w6676, element="全部读取" ("元素"), error in (no error)=w6677) -> (queue out=w6680:refnum<queue>, error out=w6679:errorcluster)  [unwired: 2 out]
                      }
                    }
                    n4597 = global write "EV05全局变量1.vi" "写入超时"(w6656) -> ()
                    n4598 = global write "EV05全局变量1.vi" "流控帧"(w6656) -> ()
                    n4599 = local write "写?"(w6656) -> ()
                    n4600 = local write "消除"(w6657) -> ()
                    n4601 = local write "控制1"(w6657) -> ()
                    n4602 = global write "EV05全局变量1.vi" "流控帧 2"(w6657) -> ()
                  }
                }
              }
            }
          }
          event "开启均衡": Value Change {
            n4603 = event-data() -> ("NewVal"=w6686:bool)  [unwired: 5 out]
            n4604 = case shown="真" w6686 {
              tunnel: w6685 -> [w6688 w6695]
              tunnel: w6684 -> [w6687 w6694]
              tunnel: [w6688 w6693] -> w6683
              tunnel: [w6687 w6692] -> w6682
              frame False {
              }
              frame True {
                n4605 = global read "EV05全局变量1.vi" "授权功能"() -> (w6690:bool)
                n4606 = case shown="假" w6690 {
                  tunnel: [TRUE ("发送成功") w6705] -> w6691
                  frame False {
                  }
                  frame True {
                    n4607 = local read "主从选择"() -> (w6697:enum32{"主板", "从板"})
                    n4608 = case shown="\"从板\"" w6697 {
                      tunnel: [0.0 ("FUNC") w6707] -> w6698
                      frame "主板", Default {
                      }
                      frame "从板" {
                        n4609 = local read "从板号"() -> (w6707:u8)
                      }
                    }
                    n4610 = local read "设备索引号"() -> (w6700:u16)
                    n4611 = local read "CAN卡类型"() -> (w6701:u32)
                    n4612 = local read "CAN端口"() -> (w6699:u16)
                    n4613 = call "标定授权发送.vi"("CAN卡类型"=w6701, "解锁类型"=enum16{"读取", "写", "下载"}."写", "设备索引号"=w6700, "CAN端口"=w6699, "是否连接"=TRUE, "板选择"=0, "FUNC"=w6698) -> ("发送成功"=w6705:bool)  [unwired: 8 out]
                  }
                }
                n4614 = case shown="真" w6691 {
                  tunnel: w6695 -> [w6709 w6714]
                  tunnel: w6694 -> [w6708 w6713]
                  tunnel: [w6709 w6711] -> w6693
                  tunnel: [w6708 w6710] -> w6692
                  frame False {
                  }
                  frame True {
                    n4615 = Enqueue Element(queue=w6714, element="开启均衡" ("元素"), error in (no error)=w6713) -> (queue out=w6711:refnum<queue>, error out=w6710:errorcluster)  [unwired: 2 out]
                  }
                }
                n4616 = call <vilib>:"Set Busy.vi"("disable click? (T)"=TRUE) -> ()  [unwired: 3 in, 8 out]
              }
            }
          }
          event "关闭均衡": Value Change {
            n4617 = event-data() -> ("NewVal"=w6719:bool)  [unwired: 5 out]
            n4618 = case shown="真" w6719 {
              tunnel: w6718 -> [w6721 w6728]
              tunnel: w6717 -> [w6720 w6727]
              tunnel: [w6721 w6726] -> w6716
              tunnel: [w6720 w6725] -> w6715
              frame False {
              }
              frame True {
                n4619 = global read "EV05全局变量1.vi" "授权功能"() -> (w6723:bool)
                n4620 = case shown="假" w6723 {
                  tunnel: [TRUE ("发送成功") w6738] -> w6724
                  frame False {
                  }
                  frame True {
                    n4621 = local read "主从选择"() -> (w6730:enum32{"主板", "从板"})
                    n4622 = case shown="\"从板\"" w6730 {
                      tunnel: [0.0 ("FUNC") w6740] -> w6731
                      frame "主板", Default {
                      }
                      frame "从板" {
                        n4623 = local read "从板号"() -> (w6740:u8)
                      }
                    }
                    n4624 = local read "设备索引号"() -> (w6733:u16)
                    n4625 = local read "CAN卡类型"() -> (w6734:u32)
                    n4626 = local read "CAN端口"() -> (w6732:u16)
                    n4627 = call "标定授权发送.vi"("CAN卡类型"=w6734, "解锁类型"=enum16{"读取", "写", "下载"}."写", "设备索引号"=w6733, "CAN端口"=w6732, "是否连接"=TRUE, "板选择"=0, "FUNC"=w6731) -> ("发送成功"=w6738:bool)  [unwired: 8 out]
                  }
                }
                n4628 = case shown="真" w6724 {
                  tunnel: w6728 -> [w6742 w6747]
                  tunnel: w6727 -> [w6741 w6746]
                  tunnel: [w6742 w6744] -> w6726
                  tunnel: [w6741 w6743] -> w6725
                  frame False {
                  }
                  frame True {
                    n4629 = Enqueue Element(queue=w6747, element="关闭均衡" ("元素"), error in (no error)=w6746) -> (queue out=w6744:refnum<queue>, error out=w6743:errorcluster)  [unwired: 2 out]
                  }
                }
                n4630 = call <vilib>:"Set Busy.vi"("disable click? (T)"=TRUE) -> ()  [unwired: 3 in, 8 out]
              }
            }
          }
          event "强制开启均衡": Value Change {
            n4631 = event-data() -> ("NewVal"=w6752:bool)  [unwired: 5 out]
            n4632 = case shown="真" w6752 {
              tunnel: w6751 -> [w6754 w6761]
              tunnel: w6750 -> [w6753 w6760]
              tunnel: [w6754 w6759] -> w6749
              tunnel: [w6753 w6758] -> w6748
              frame False {
              }
              frame True {
                n4633 = global read "EV05全局变量1.vi" "授权功能"() -> (w6756:bool)
                n4634 = case shown="假" w6756 {
                  tunnel: [TRUE ("发送成功") w6771] -> w6757
                  frame False {
                  }
                  frame True {
                    n4635 = local read "主从选择"() -> (w6763:enum32{"主板", "从板"})
                    n4636 = case shown="\"从板\"" w6763 {
                      tunnel: [0.0 ("FUNC") w6773] -> w6764
                      frame "主板", Default {
                      }
                      frame "从板" {
                        n4637 = local read "从板号"() -> (w6773:u8)
                      }
                    }
                    n4638 = local read "设备索引号"() -> (w6766:u16)
                    n4639 = local read "CAN卡类型"() -> (w6767:u32)
                    n4640 = local read "CAN端口"() -> (w6765:u16)
                    n4641 = call "标定授权发送.vi"("CAN卡类型"=w6767, "解锁类型"=enum16{"读取", "写", "下载"}."写", "设备索引号"=w6766, "CAN端口"=w6765, "是否连接"=TRUE, "板选择"=0, "FUNC"=w6764) -> ("发送成功"=w6771:bool)  [unwired: 8 out]
                  }
                }
                n4642 = case shown="真" w6757 {
                  tunnel: w6761 -> [w6775 w6780]
                  tunnel: w6760 -> [w6774 w6779]
                  tunnel: [w6775 w6777] -> w6759
                  tunnel: [w6774 w6776] -> w6758
                  frame False {
                  }
                  frame True {
                    n4643 = Enqueue Element(queue=w6780, element="强制均衡" ("元素"), error in (no error)=w6779) -> (queue out=w6777:refnum<queue>, error out=w6776:errorcluster)  [unwired: 2 out]
                  }
                }
                n4644 = call <vilib>:"Set Busy.vi"("disable click? (T)"=TRUE) -> ()  [unwired: 3 in, 8 out]
              }
            }
          }
        }
        n4645 = Unbundle By Name(w4005) -> ("status"=w4004:bool)
        n4646 = Or(x=w4004, y=w4006) -> (x .or. y?=w4007:bool)
      }
      n4647 = Release Queue(queue=w4001, force destroy? (F)=TRUE ("强制销毁？(F)"), error in (no error)=w4000) -> (error out=w3998:errorcluster)  [unwired: 2 out]
      n4648 = call <vilib>:"Clear Errors.vi"("error in (no error)"=w3998) -> ()  [unwired: 7 out]
    }
    frame Enabled {
    }
  }
  n4649 = Release Queue(queue=w34, force destroy? (F)=TRUE ("强制销毁？(F)"), error in (no error)=w33) -> (error out=w36:errorcluster)  [unwired: 2 out]
  n4650 = call <vilib>:"Clear Errors.vi"("error in (no error)"=w36) -> ()  [unwired: 7 out]
  n4651 = local write "面板选择"(T7."读写参数" ("面板选择")) -> ()
  n4652 = local write "停止"(FALSE ("退出？(T)")) -> ()
